vi "Exercise1.vi"   [LabVIEW 2014, in "Brandon_5th.lvrbt"]
uses:
  Brandon_5th.lvrbt
  <vilib>/NXT/Block Support/NXT_OutputPort.ctl
  <vilib>/NXT/NXTIO Xnodes/NXTIONodeSubVIs/NXTMoveMotors.vi
  <vilib>/NXT/Dual Mode Library/Waits/Wait_Num.vi
  <vilib>/NXT/Subs/LVHSConnector.ctl
  <vilib>/NXT/NXTIO Xnodes/AddressXNode/NXTIOAddress.xnode
  <vilib>/NXT/NXTIO Xnodes/NXTIOXNode/NXTIO.xnode
  <vilib>/NXT/LegoClasses/BrickReference/BrickReference.lvclass
types:
  T1 = typedef "NXT_OutputPort.ctl" = u8
  T2 = typedef "LVHSConnector.ctl" = refnum<class "BrickReference.lvclass">
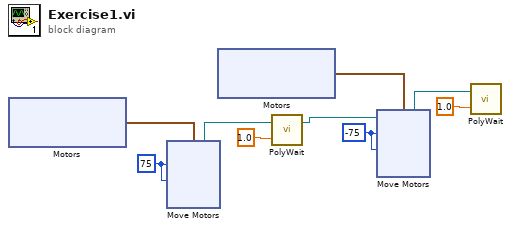
[diagram p0: block diagram]
diagram:
  w3 = i8 -75 ("Power/Speed 1")
  w7 = i8 75 ("Power/Speed 1")
  n1 = xnode "Motors"() -> ("Motor"=w8:cluster{"Port":T1, "Port":T1})
  n2 = xnode "Move Motors"("Power/Speed 2"=w7, "Power/Speed 1"=w7, "Motors"=w8) -> ("NXT/EV3"=w9:T2)  [unwired: 1 in]
  n3 = xnode "Motors"() -> ("Motor"=w4:cluster{"Port":T1, "Port":T1})
  n4 = call-poly <vilib>:"PolyWait.vi"("Time (1 sec)"=sgl 1.0, "NXT/EV3"=w9) -> ("NXT/EV3"=w1:T2)  [unwired: 2 in]
  n5 = xnode "Move Motors"("Power/Speed 2"=w3, "Power/Speed 1"=w3, "Motors"=w4, "NXT/EV3"=w1) -> ("NXT/EV3"=w5:T2)
  n6 = call-poly <vilib>:"PolyWait.vi"("Time (1 sec)"=sgl 1.0, "NXT/EV3"=w5) -> ()  [unwired: 2 in, 1 out]
